vi "XYZStage-Direct move.vi"(10 "Current State":T1, 11 "Coordinate to set":enum16{"X", "Y", "Z"}(ring)) -> (1 "Timed out while waiting for acknowledgement":bool, 2 "Acknowledgement message":string)   [LabVIEW 2017]
uses:
  User Interface/Windows/Position control window/Typedefs/Pos Ctrl States.ctl
  User Interface/Windows/Position control window/Globals/Pos ctrl window globals.vi
panel:
  out "Wait for acknowledge?":bool
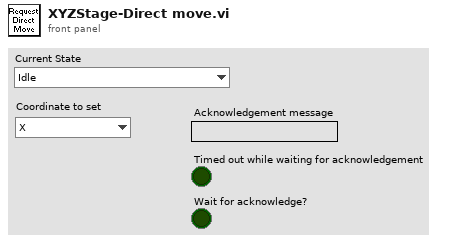
[diagram p1: front panel]
types:
  T1 = typedef "Pos Ctrl States.ctl" = enum16{"Idle", "Count-down", "Request single step (ack.)", "Request single step (no ack.)", "Request continuous movement", "Request movement stop"}
  T2 = typedef "Pos Ctrl window refs cluster.ctl" = cluster{"menu reference":refnum<k9>, "X Coordinate ctrl":refnum<vi>, "Y Coordinate ctrl":refnum<vi>, "Z Coordinate ctrl":refnum<vi>, "Speed setting ctrl":refnum<vi>, "Up":refnum<vi>, "Down":refnum<vi>, "Left":refnum<vi>, "Right":refnum<vi>, "Z move up":refnum<vi>, "Z move down":refnum<vi>, "Down-left":refnum<vi>, "Down-right":refnum<vi>, "Up-left":refnum<vi>, "Up-right":refnum<vi>, "Step = size of image":refnum<vi>, "XY step (um)":refnum<vi>, "Z step (um)":refnum<vi>}
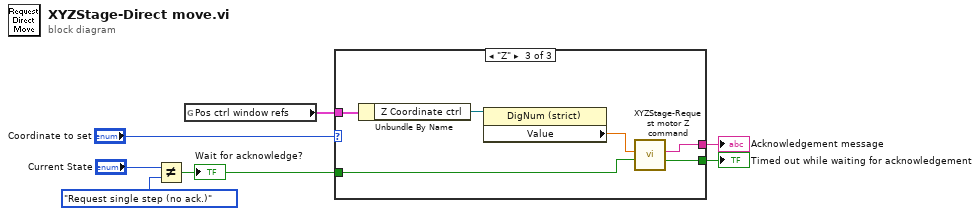
[diagram p0: block diagram]
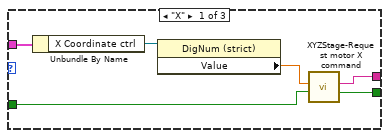
[diagram p2: hidden frame]
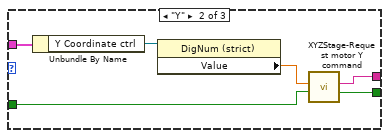
[diagram p3: hidden frame]
diagram:
  n1 = Not Equal?(x="Current State", y=Pos_Ctrl_States."Request single step (no ack.)" ("x")) -> (x != y?=w1:bool)
  "Wait for acknowledge?" <- w1
  n2 = global read "Pos ctrl window globals.vi" "Pos ctrl window refs"() -> (w6:T2)
  n3 = case shown="\"Z\"" "Coordinate to set" {
    tunnel: w6 -> [w13 w19 w25]
    tunnel: [w10 w16 w22] -> w5
    tunnel: [w9 w15 w21] -> w4
    tunnel: w1 -> [w8 w14 w20]
    frame "X" {
      n4 = Unbundle By Name(w13) -> ("X Coordinate ctrl"=w12:refnum<vi>)
      n5 = property class="DigNum (strict)"(reference=w12) -> ("Value"=w11:sgl)  [unwired: 1 in, 2 out]
      n6 = call "XYZStage-Request motor X command.vi"("Wait for acknowledge?"=w8, "Motor X"=w11) -> ("Timed out while waiting for acknowledgement"=w9:bool, "Acknowledgement message"=w10:string)  [unwired: 8 in]
    }
    frame "Y" {
      n7 = Unbundle By Name(w19) -> ("Y Coordinate ctrl"=w18:refnum<vi>)
      n8 = property class="DigNum (strict)"(reference=w18) -> ("Value"=w17:sgl)  [unwired: 1 in, 2 out]
      n9 = call "XYZStage-Request motor Y command.vi"("Wait for acknowledge?"=w14, "Motor Y"=w17) -> ("No acknowledgement"=w15:bool, "Acknowledgement message"=w16:string)  [unwired: 8 in]
    }
    frame "Z" {
      n10 = Unbundle By Name(w25) -> ("Z Coordinate ctrl"=w24:refnum<vi>)
      n11 = property class="DigNum (strict)"(reference=w24) -> ("Value"=w23:sgl)  [unwired: 1 in, 2 out]
      n12 = call "XYZStage-Request motor Z command.vi"("Wait for acknowledge?"=w20, "Motor Z"=w23) -> ("Timed out while waiting for acknowledgement"=w21:bool, "Acknowledgement message"=w22:string)  [unwired: 7 in, 1 out]
    }
  }
  "Timed out while waiting for acknowledgement" <- w4
  "Acknowledgement message" <- w5
